vi "Plate Assignment Parse.vi"(10 "Game String":string, 11 "Plate Arrangement":T1) -> (3 "Match?":bool)   [LabVIEW 2019]
uses:
  AutonBuilder/Typedef/Plate Arrangement.ctl
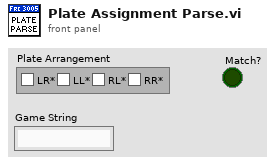
[diagram p1: front panel]
types:
  T1 = typedef "Plate Arrangement.ctl" = cluster{"LR*":bool, "LL*":bool, "RL*":bool, "RR*":bool}
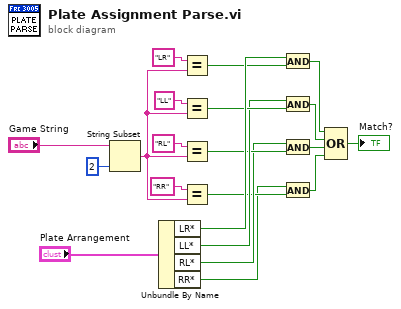
[diagram p0: block diagram]
diagram:
  n1 = String Subset(string="Game String", length (rest)=2 ("length (rest)")) -> (substring=w12:string)  [unwired: 1 in]
  n2 = Unbundle By Name("Plate Arrangement") -> ("LR*"=w21:bool, "LL*"=w10:bool, "RL*"=w8:bool, "RR*"=w6:bool)
  n3 = Equal?(x="LR", y=w12) -> (x = y?=w20:bool)
  n4 = Equal?(x="LL", y=w12) -> (x = y?=w11:bool)
  n5 = Equal?(x="RL", y=w12) -> (x = y?=w9:bool)
  n6 = Equal?(x="RR", y=w12) -> (x = y?=w7:bool)
  n7 = And(x=w21, y=w20) -> (x .and. y?=w5:bool)
  n8 = And(x=w10, y=w11) -> (x .and. y?=w4:bool)
  n9 = And(x=w8, y=w9) -> (x .and. y?=w3:bool)
  n10 = And(x=w6, y=w7) -> (x .and. y?=w2:bool)
  n11 = Compound Arithmetic op=OR(w5, w4, w3, w2) -> (→"Match?":bool)
